vi "change alarm comparison data type.vi"(7 "data type":T1, 8 "error in":errorcluster, 9 "compare index":i32, 10 "alarm name":string, 11 "alarms module configuration in":refnum<class "alarms module configuration.lvclass">) -> (0 "error out":errorcluster, 2 "changed channel":refnum<class "TBM channel.lvclass">[](array[class]), 3 "alarms module configuration out":refnum<class "alarms module configuration.lvclass">)   [LabVIEW 2013, in "alarms module configuration.lvclass"]
uses:
  alarms module configuration.lvclass
  <vilib>/NI/Tag Bus/tag/Data Type.ctl
  <vilib>/NI/Tag Bus Module Framework/channel/TBM channel.lvclass
  alarms module configuration.lvclass/alarms module configuration.ctl
  <vilib>/NI/Tag Bus/tag/tag descriptor.lvclass/tag descriptor.ctl
  <vilib>/NI/Tag Bus/tag/tag descriptor.lvclass
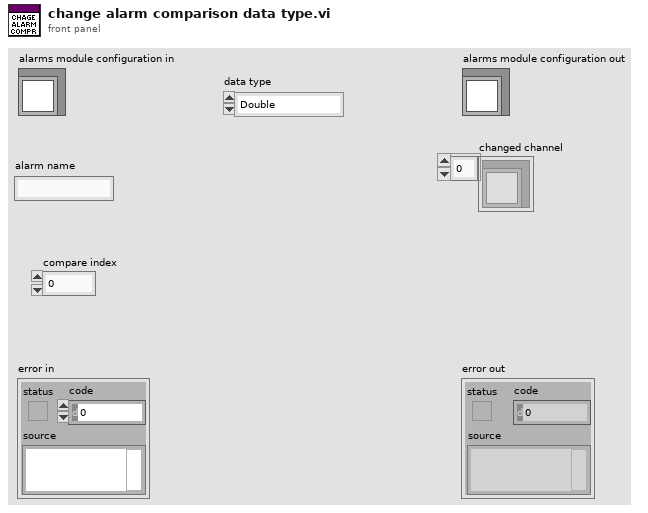
[diagram p1: front panel]
types:
  T1 = typedef "tag bus.lvlib/tag descriptor.lvclass/Data Type.ctl" = enum16{"Double", "Single", "I64", "I32", "I16", "I8", "U64", "U32", "U16", "U8", "Boolean", "String", "Array of Double", "Array of Single", "Array of I64", "Array of I32", "Array of I16", "Array of I8", "Array of U64", "Array of U32", "Array of U16", "Array of U8", "Array of Boolean", "Array of String"}
  T2 = typedef "alarms module configuration.lvclass/alarm configuration.ctl" = cluster{"alarm name":string, "comparisons":T3[], "unlatch":refnum<class "TBM channel.lvclass">, "output":refnum<class "TBM channel.lvclass">, "boolean op":T5}
  T3 = typedef "alarms module configuration.lvclass/alarm comparison.ctl" = cluster{"input channel":refnum<class "TBM channel.lvclass">, "limit":dbl, "comparison":T4}
  T4 = typedef "alarms module configuration.lvclass/compare type.ctl" = enum16{">", "<", ">=", "<=", "="}
  T5 = typedef "alarms module configuration.lvclass/boolean operation.ctl" = enum16{"AND", "OR"}
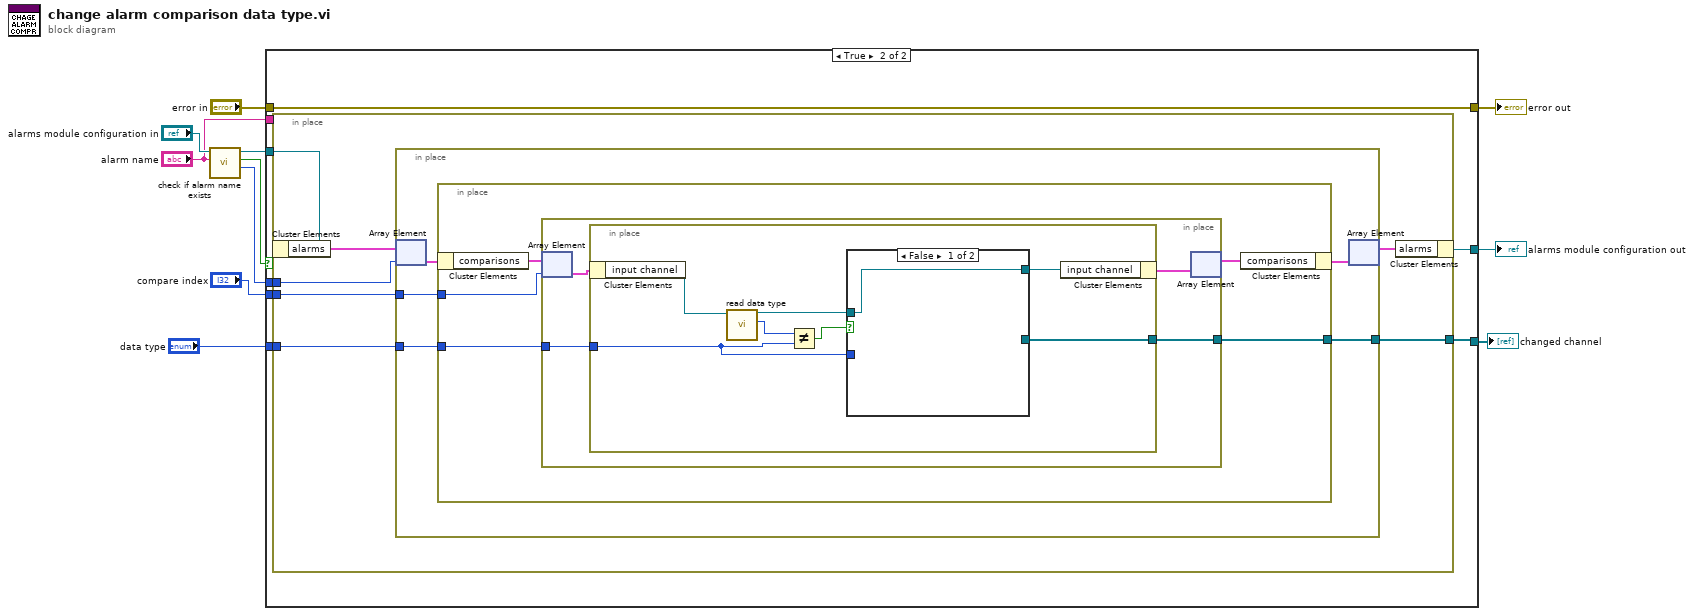
[diagram p0: block diagram]
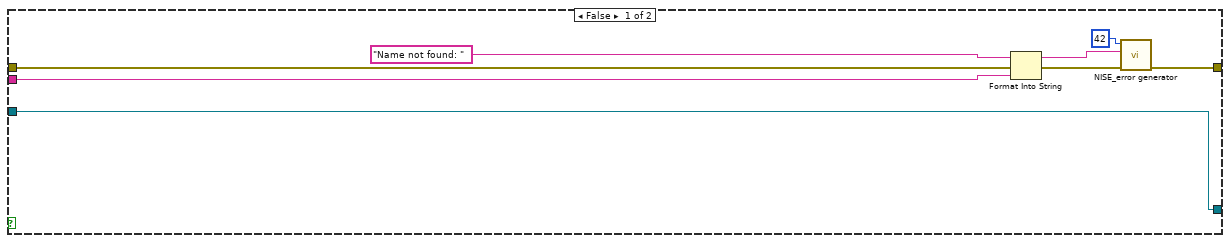
[diagram p2: hidden frame]
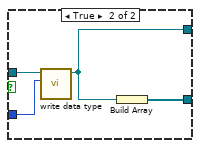
[diagram p3: hidden frame]
diagram:
  n1 = call "check if alarm name exists.vi"("name to locate"="alarm name", "alarms module configuration in"="alarms module configuration in") -> ("index"=w5:i32, "found?"=w8:bool, "alarms module configuration out"=w6:refnum<class "alarms module configuration.lvclass">)  [unwired: 6 in, 1 out]
  n2 = case shown="True" w8 {
    tunnel: [w18 w24] -> w10
    tunnel: "error in" -> [w19 w24]
    tunnel: [w13 w25] -> w7
    tunnel: w6 -> [w13 w26]
    tunnel: w5 -> [_ w23]
    tunnel: "alarm name" -> [w12 _]
    tunnel: "compare index" -> [_ w22]
    tunnel: "data type" -> [_ w21]
    tunnel: [_ w20] -> w1
    frame False {
      n3 = Format Into String(initial string="Name not found: " ("append error message"), error in=w19, w12) -> (resulting string=w14:string, error out=w16:errorcluster)  [unwired: 1 in]
      n4 = call <vilib>:"NISE_error generator.vi"("error in"=w16, "append error message"=w14, "error code (0)"=42) -> ("error out"=w18:errorcluster)  [unwired: 6 in]
    }
    frame True {
      n5 = in-place {
        in-place-border: w23 -> [w30]
        in-place-border: w22 -> [w29]
        in-place-border: w21 -> [w28]
        in-place-border: [w27] -> w20
        n6 = in-place-cluster #1(w26) -> ("alarms"=w32:T2[])
        n7 = in-place {
          in-place-border: w29 -> [w36]
          in-place-border: w28 -> [w34]
          in-place-border: [w33] -> w27
          n8 = in-place-array #2(w32, w30) -> (w37:T2)
          n9 = in-place {
            in-place-border: w36 -> [w40]
            in-place-border: w34 -> [w39]
            in-place-border: [w38] -> w33
            n10 = in-place-cluster #3(w37) -> ("comparisons"=w42:T3[])
            n11 = in-place {
              in-place-border: w39 -> [w44]
              in-place-border: [w43] -> w38
              n12 = in-place-array #4(w42, w40) -> (w46:T3)
              n13 = in-place {
                in-place-border: w44 -> [w49]
                in-place-border: [w47] -> w43
                n14 = in-place-cluster #5(w46) -> ("input channel"=w52:refnum<class "TBM channel.lvclass">)
                n15 = call <vilib>:"read data type.vi"("system tag in"=w52) -> ("data type"=w53:T1, "system tag out"=w50:refnum<class "TBM channel.lvclass">)  [unwired: 8 in, 1 out]
                n16 = Not Equal?(x=w53, y=w49) -> (x != y?=w51:bool)
                n17 = case shown="False" w51 {
                  tunnel: w50 -> [w54 w58]
                  tunnel: [w54 w56] -> w48
                  tunnel: w49 -> [_ w57]
                  tunnel: [_ w55] -> w47
                  frame False {
                  }
                  frame True {
                    n18 = call <vilib>:"write data type.vi"("data type"=w57, "system tag in"=w58) -> ("system tag out"=w56:refnum<class "TBM channel.lvclass">)  [unwired: 8 in, 1 out]
                    n19 = Build Array(w56) -> (w55:refnum<class "TBM channel.lvclass">[])
                  }
                }
                n20 = in-place-cluster #5("input channel"=w48) -> (w45:T3)
              }
              n21 = in-place-array #4(w45) -> (w41:T3[])  [unwired: 1 out]
            }
            n22 = in-place-cluster #3("comparisons"=w41) -> (w35:T2)
          }
          n23 = in-place-array #2(w35) -> (w31:T2[])  [unwired: 1 out]
        }
        n24 = in-place-cluster #1("alarms"=w31) -> (w25:refnum<class "alarms module configuration.lvclass">)
      }
    }
  }
  "error out" <- w10
  "alarms module configuration out" <- w7
  "changed channel" <- w1
